vi "serial robot.vi"(0 "Numeric":dbl, 1 "Numeric 2":dbl, 2 "Numeric 3":dbl, 3 "Numeric 4":dbl) -> ()   [LabVIEW 2010]
doc: "The Basic Serial Read and Write example performs a Serial Port Read, a Serial Port Write, or a combination of these actions. The user selects the actions (read or write) on the front panel. If both are selected, the VI will write the data first, read data, and then close the VISA session that is opened to the port. This VI will wait until the specified number of bytes is received at the port or until a termination character is read.\n\nINSTRUCTIONS:\n1) Select the serial resource and configuration parameters (baud rate, data bits, parity, stop bits, flow control).\n2) Select the operations to be performed. \n3) Connect the serial port to your device. If no device is available, perform a loopback test by doing one of the following. Short pins 2 and 3 on a RS-232 cable or short pin 4 to pin 8 and pin 5 to pin 9 on a RS-485/422 cable. \n4) Run the VI to see the data read. (The \"read string\" will match the \"string to write\" if a loopback test was performed.)\n\nNote: The parameters set for the serial port must match the parameters of the connected instrument or device. In this example, the bytes to read parameter specifies the number of bytes that the serial port reads. If there were more bytes at the port than the number specified in bytes to read, those bytes would not be read. Also, if you specify to read more bytes than the number of bytes actually read, you might receive a timeout error message.\n\nOn the block diagram, the Configure Serial Port VI sets the configuration parameters. The front panel displays the controls used to configure the basic parameters, such as baud rate, data bits, and parity. Constants configure the other parameters the user probably does not need set. After the VISA Configure Serial Port VI opens the VISA session and configures the port, the VI passes the VISA resource name to other VIs that perform operations on that VISA resource. The VISA Write function sends a command to the serial device and the VISA Read function returns data based on the command. The VISA Close function then closes the reference to the serial device. It is important to close the reference; otherwise communication through with that port through protocols other than VISA might not be possible."
uses:
  <vilib>/Instr/_visa.llb/VISA Configure Serial Port (Instr).vi
panel:
  out "concatenated string":string
  in  "flow control":u16(ring) items=["None"=0, "XON/XOFF"=1, "RTS/CTS"=2, "DTR/DSR"=4]
  in  "stop bits":u16(ring)=10 items=["1.0"=10, "1.5"=15, "2.0"=20]
  in  "parity":u16(ring) items=["None", "Odd", "Even", "Mark", "Space"]
  in  "data bits":u16=8 min=5 max=8 step=1
  in  "VISA resource name":refnum<visa-resource-name>="COM1"
  out "Numeric 7":i32
  out "substring 3":string
  in  "write button":bool
  in  "MOTOR SELECTION SWITCH":i32(knob) scale=0.0..5.0
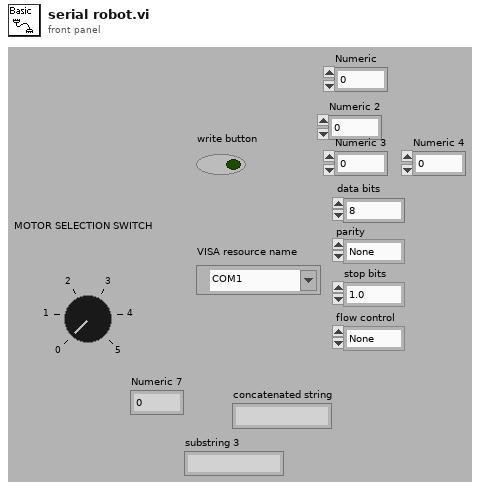
[diagram p1: front panel]
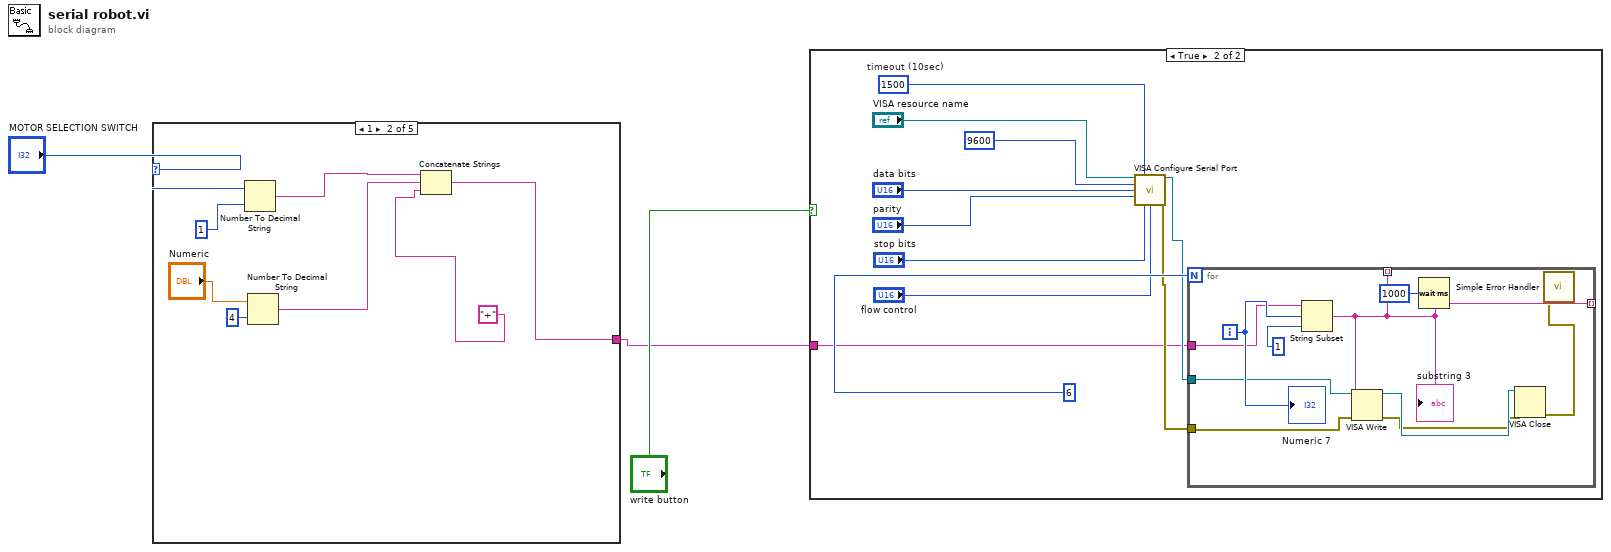
[diagram p0: block diagram]
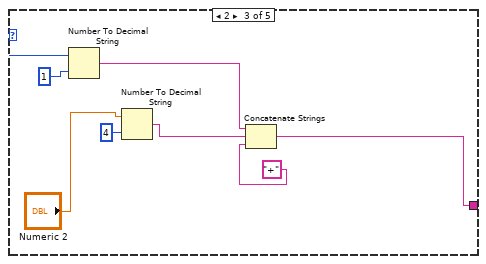
[diagram p4: hidden frame]
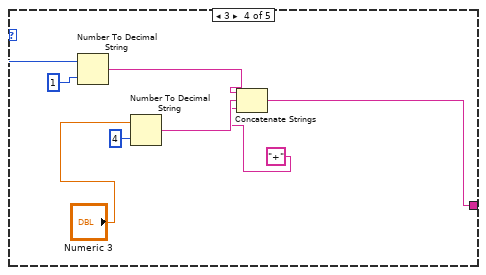
[diagram p5: hidden frame]
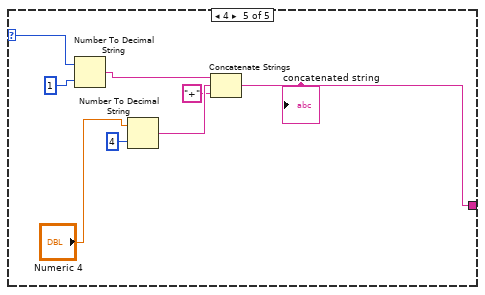
[diagram p6: hidden frame]
diagram:
  n1 = case shown="1" "MOTOR SELECTION SWITCH" {
    selector: "MOTOR SELECTION SWITCH" -> [_ w10 w18 w26 w34]
    tunnel: [_ w5 w13 w21 w29] -> w1
    frame 0, Default {
    }
    frame 1 {
      n2 = Number To Decimal String(number=w10, width (-)=i16 1) -> (decimal integer string=w7:string)
      n3 = Number To Decimal String(number="Numeric", width (-)=i16 4) -> (decimal integer string=w6:string)
      n4 = Concatenate Strings(w7, w6, "+" ("string")) -> (w5:string)
    }
    frame 2 {
      n5 = Number To Decimal String(number=w18, width (-)=i16 1) -> (decimal integer string=w14:string)
      n6 = Number To Decimal String(number="Numeric 2", width (-)=i16 4) -> (decimal integer string=w15:string)
      n7 = Concatenate Strings(w14, w15, "+" ("string")) -> (w13:string)
    }
    frame 3 {
      n8 = Number To Decimal String(number=w26, width (-)=i16 1) -> (decimal integer string=w23:string)
      n9 = Number To Decimal String(number="Numeric 3", width (-)=i16 4) -> (decimal integer string=w22:string)
      n10 = Concatenate Strings(w23, w22, "+" ("string")) -> (w21:string)
    }
    frame 4 {
      n11 = Number To Decimal String(number=w34, width (-)=i16 1) -> (decimal integer string=w30:string)
      n12 = Number To Decimal String(number="Numeric 4", width (-)=i16 4) -> (decimal integer string=w31:string)
      n13 = Concatenate Strings(w30, w31, "+" ("string")) -> (w29:string)
      "concatenated string" <- w29
    }
  }
  n14 = case shown="True" "write button" {
    tunnel: w1 -> [_ w36]
    frame False {
    }
    frame True {
      w41 = u32 1500  # timeout (10sec)
      n15 = call-poly "VISA Configure Serial Port"("VISA resource name"="VISA resource name", "timeout (10sec)"=w41, "baud rate (9600)"=u32 9600 ("baud rate"), "data bits (8)"="data bits", "parity (0:none)"="parity", "stop bits (10: 1 bit)"="stop bits", "flow control (0:none)"="flow control") -> ("VISA resource name out"=w37:refnum<visa-resource-name>, "error out"=w38:errorcluster)  [unwired: 2 in, 5 out]
      n16 = for {
        N: 6 -> [_]
        tunnel: [w54] -> _ mode=indexing
        tunnel: [w54] -> _ mode=indexing
        tunnel: w38 -> [w52]
        tunnel: w37 -> [w51]
        tunnel: w36 -> [w50]
        i -> [w56]
        n17 = String Subset(string=w50, offset (0)=w56, length (rest)=1 ("length (rest)")) -> (substring=w54:string)
        "substring 3" <- w54
        n18 = VISA Write(VISA resource name=w51, write buffer=w54, error in (no error)=w52) -> (VISA resource name out=w49:refnum<visa-resource-name>, error out=w48:errorcluster)  [unwired: 1 out]
        n19 = Wait (ms)(milliseconds to wait=u32 1000) -> ()  [unwired: 1 out]
        n20 = VISA Close(VISA resource name=w49, error in (no error)=w48) -> (error out=w53:errorcluster)
        n21 = call <vilib>:"Simple Error Handler.vi"("error in (no error)"=w53) -> ()  [unwired: 1 in, 8 out]
        "Numeric 7" <- w56
      }
    }
  }
